vi "WAIT_FOR_DATA.vi"(10 "argv":string[](array[string]), 11 "args":u8) -> ()   [LabVIEW 2011]
uses:
  signals/Signal.ctl
  2012vision/Camera State.ctl
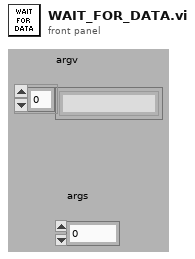
[diagram p1: front panel]
types:
  T1 = typedef "Signal.ctl" = enum16{"SIGFIRE", "SIGSTOPSCRIPT", "SIGSTARTGUN", "SIGSTOPGUN", "SIGDISABLED", "SIGENABLED", "SIGUDPTIMEOUT", "SIGNEWVISION_REMOTE", "SIGNEWVISION_LOCAL", "SIGSHOTFIRED", "SIGDOTRACK", "SIGDONTTRACK"}
  T2 = enum16{"Get Latest Data", "Get Local Data", "Get Remote Data", "Set Local Data", "Set Remote Data"}
  T3 = typedef "Camera State.ctl" = enum16{"No Targets", "Low Confidence", "Medium Confidence", "High Confidence", "Camera Error"}
  T4 = cluster{"X Position":dbl, "Distance":dbl, "Camera State":T3}
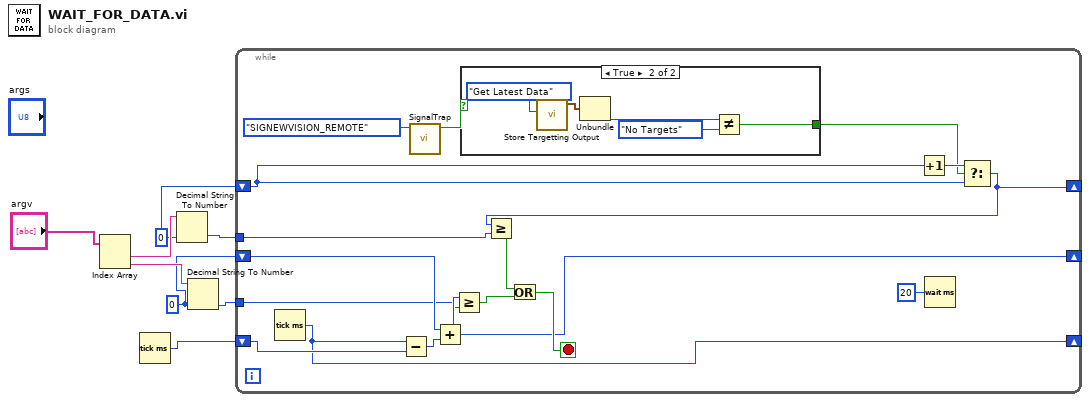
[diagram p0: block diagram]
diagram:
  w4 = u32 0 ("default (0 I32)")
  w3 = 0 ("default (0 I32)")
  n1 = Index Array(array="argv") -> (element #1=w7:string, element #2=w6:string)  [unwired: 2 in]
  n2 = Tick Count (ms)() -> (millisecond timer value=w1:u32)
  n3 = Decimal String To Number(string=w7, default (0L)=w3) -> (number=w2:i32)  [unwired: 1 in, 1 out]
  n4 = Decimal String To Number(string=w6, default (0L)=w4) -> (number=w5:u32)  [unwired: 1 in, 1 out]
  n5 = while {
    shift-right: [w18] -> _
    shift-left: w3 -> [w14]
    shift-right: [w22] -> _
    shift-left: w4 -> [w25]
    tunnel: w5 -> [w21]
    tunnel: w2 -> [w17]
    shift-right: [w12] -> _
    shift-left: w1 -> [w13]
    stop <- w23 stop-if-true
    n6 = Tick Count (ms)() -> (millisecond timer value=w12:u32)
    n7 = Subtract(x=w12, y=w13) -> (x-y=w24:u32)
    n8 = call "SignalTrap.vi"("Signal"=Signal."SIGNEWVISION_REMOTE") -> ("Trapped Signal"=w11:bool)  [unwired: 10 in]
    n9 = Add(x=w25, y=w24) -> (x+y=w22:u32)
    n10 = Greater Or Equal?(x=w22, y=w21) -> (x >= y?=w20:bool)
    n11 = case shown="True" w11 {
      selector: w11 -> [w26 _]
      tunnel: [w26 w29] -> w10
      frame False {
      }
      frame True {
        n12 = call "Store Targetting Output.vi"("mode"=T2."Get Latest Data") -> ("Targetting Output"=w28:T4)  [unwired: 10 in]
        n13 = Unbundle(w28) -> ("Camera State"=w31:T3)  [unwired: 2 out]
        n14 = Not Equal?(x=w31, y=Camera_State."No Targets") -> (x != y?=w29:bool)
      }
    }
    n15 = Increment(x=w14) -> (x+1=w15:i32)
    n16 = Wait (ms)(milliseconds to wait=u32 20) -> ()  [unwired: 1 out]
    n17 = Select(t=w15, s=w10, f=w14) -> (s? t:f=w18:i32)
    n18 = Greater Or Equal?(x=w18, y=w17) -> (x >= y?=w16:bool)
    n19 = Or(x=w16, y=w20) -> (x .or. y?=w23:bool)
  }
